vi "GetDetectPosWithDispDotPos.vi"(3 "返回值":sgl, 7 "闸门序号":i32, 8 "错误输入（无错误）":errorcluster, 9 "显示点分频时间":u16, 10 "显示点位置":u16, 11 "需要转换的通道":u8) -> (0 "错误输出":errorcluster)   [LabVIEW 2014]
uses:
  ZXUTConfigMgr.dll
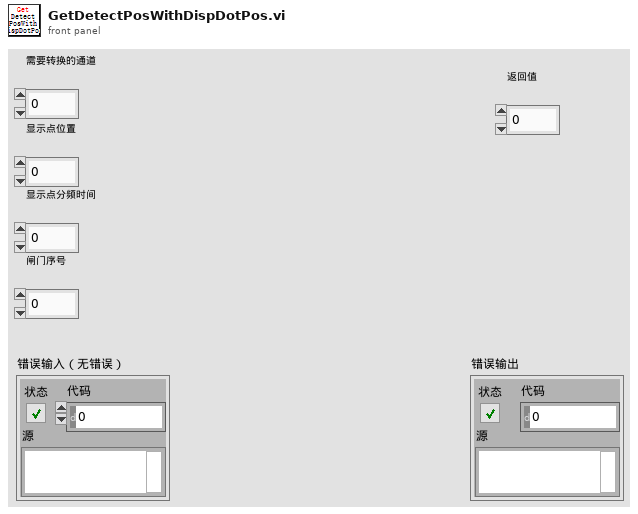
[diagram p1: front panel]
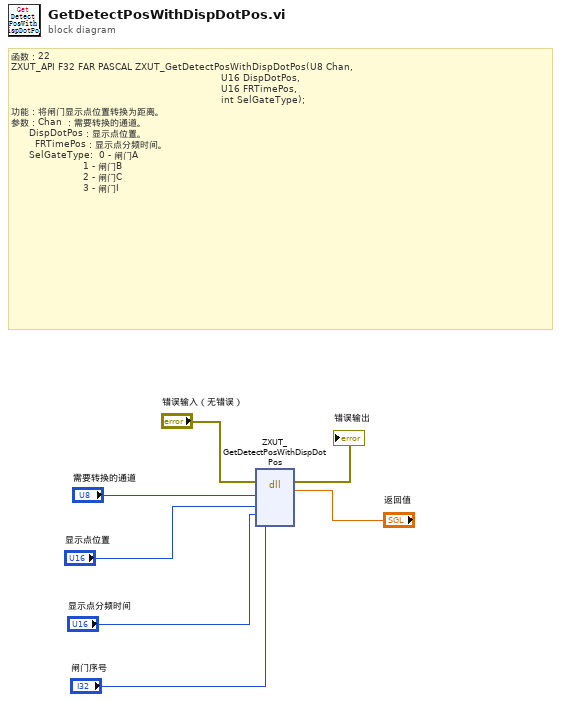
[diagram p0: block diagram]
diagram:
  # "函数：22\nZXUT_API F32\tFAR PASCAL ZXUT_GetDetectPosWithDispDotPos(U8 Chan, \n                                                                      U16 DispDotPos, \n                                                                      U16 FRTimePos,\n                                                                      int SelGateType);\n功能：将闸门显示点位置转换为距离。\n参数：Chan ：需要转换的通道。\n      DispDotPos：显示点位置。\n        FRTimePos：显示点分频时间。\n      SelGateType:  0 - 闸门A \n                        1 - 闸门B\n                        2 - 闸门C\n                        3 - 闸门I"
  n1 = dll-call lib="PTH2eabs D软件超声实时监测软件ZXUTAppDemo(华南理工V02.00)X86DllZXUTConfigMgr.dll" fn="ZXUT_GetDetectPosWithDispDotPos"(error in="错误输入（无错误）", "返回值"="返回值", "Chan"="需要转换的通道", "DispDotPos"="显示点位置", "FRTimePos"="显示点分频时间", "SelGateType"="闸门序号") -> (error out=→"错误输出":errorcluster)  [unwired: 6 in, 1 out]
